vi "Static Write.vi"(8 "error in (no error)":errorcluster, 10 "Value":dbl, 11 "Abs_Double Float in":refnum<class "Abs_Double Float.lvclass">) -> (0 "error out":errorcluster, 3 "Abs_Double Float out":refnum<class "Abs_Double Float.lvclass">)   [LabVIEW 2021, in "Abs_Double Float.lvclass"]
uses:
  Abs_Double Float.lvclass
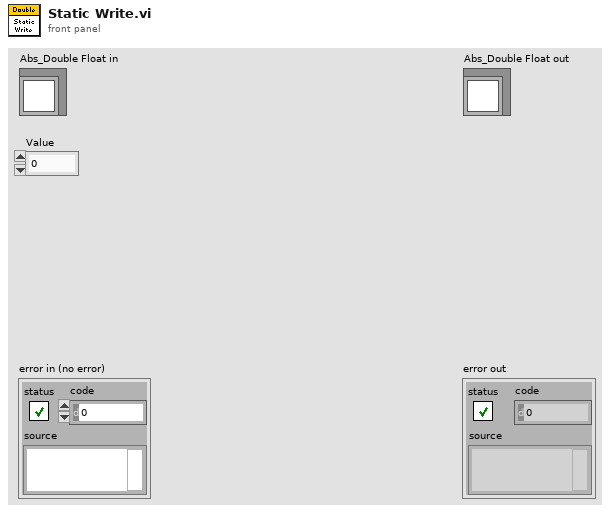
[diagram p1: front panel]
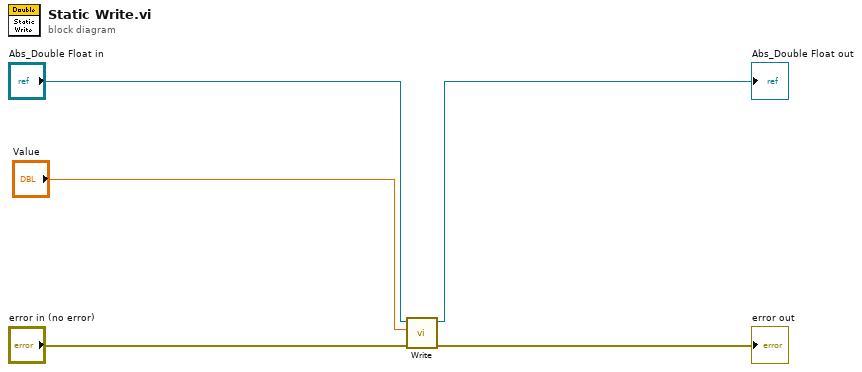
[diagram p0: block diagram]
diagram:
  n1 = call-dynamic "Write.vi"("error in (no error)"="error in (no error)", "Value"="Value", "Double Float.lvclass in"="Abs_Double Float in") -> ("error out"=→"error out":errorcluster, "Double Float.lvclass out"=→"Abs_Double Float out":refnum<class "Abs_Double Float.lvclass">)  [unwired: 7 in]
